vi "Check tree branch potential.vi"(6 "No. coins":i32, 9 "Goal amount":dbl, 10 "All my coins":dbl[](array[numeric]), 11 "Coins State Cache":bool[](array[boolean])) -> (2 "Stop?":bool, 3 "Total (£)":dbl)   [LabVIEW 2018]
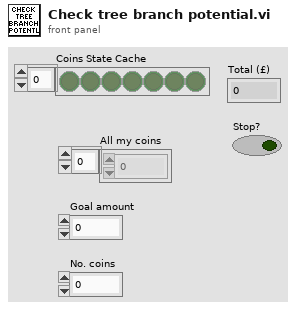
[diagram p1: front panel]
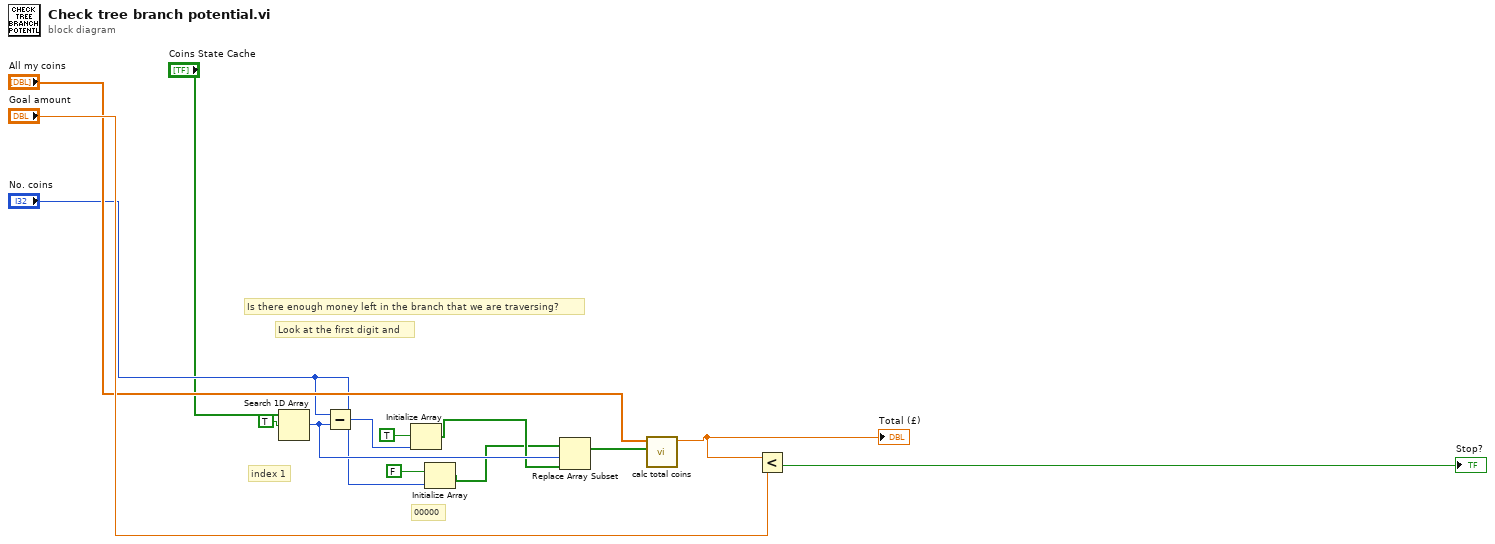
[diagram p0: block diagram]
diagram:
  # "Look at the first digit and"
  # "Is there enough money left in the branch that we are traversing?"
  # "index 1"
  # "00000"
  n1 = Search 1D Array(1D array="Coins State Cache", element=TRUE) -> (index of element=w9:i32)  [unwired: 1 in]
  n2 = Subtract(x="No. coins", y=w9) -> (x-y=w8:i32)
  n3 = Initialize Array(TRUE ("element"), w8) -> (w6:bool[])
  n4 = Initialize Array(FALSE ("element"), "No. coins") -> (w5:bool[])
  n5 = Replace Array Subset(array=w5, new element=w6, index=w9) -> (w10:bool[])
  n6 = call "calc total coins.vi"("Coins"=w10, "All my coins"="All my coins") -> ("Total (£)"=w12:dbl)  [unwired: 9 in]
  "Total (£)" <- w12
  n7 = Less?(x=w12, y="Goal amount") -> (x < y?=→"Stop?":bool)
